vi "12water.vi"() -> ()   [LabVIEW 2013]
panel:
  out "Report":string
  out "Water Level Low":bool
  out "Water Level High":bool
  in  "Water Level":dbl(slide) scale=0.0..1000.0
  out "Water Tank":dbl(slide) scale=0.0..1000.0
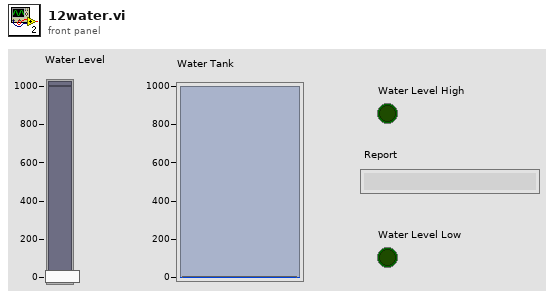
[diagram p1: front panel]
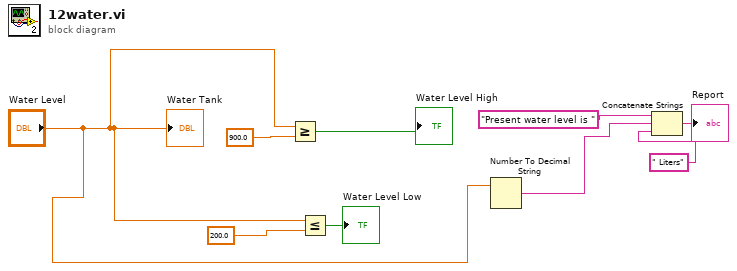
[diagram p0: block diagram]
diagram:
  n1 = Greater Or Equal?(x="Water Level", y=900.0) -> (x >= y?=→"Water Level High":bool)
  n2 = Less Or Equal?(x="Water Level", y=200.0) -> (x <= y?=→"Water Level Low":bool)
  n3 = Number To Decimal String(number="Water Level") -> (decimal integer string=w3:string)  [unwired: 1 in]
  n4 = Concatenate Strings("Present water level is " ("string"), w3, " Liters" ("string")) -> (→"Report":string)
  "Water Tank" <- "Water Level"
